vi "Main.vi"() -> ()   [LabVIEW 2014]
uses:
  <vilib>/measure/mamon.llb/Waveform Peak Detection for 1 Chan.vi
  <vilib>/measure/NI_MAPro.lvlib
panel:
  in  "Points to average":i32=50
  out "Czułość fazowa":dbl format="%#_3e"
  in  "Licz":bool
  in  "delta L [um]":dbl
  in  "L [mm]":dbl
  in  "OK Button":bool
  out "output array":dbl[](array[numeric])
  out "Locations":dbl[](array[numeric]) format="%.2p"
  in  "Reset ZOOM":bool
  out "Licznik pików":i32
  in  "stop":bool
  in  "maksimum":i32
  in  "długość przedziału":i32=100
  in  "początek przedziału":i32
  in  "próg dla maksimum":dbl format="%.2p"
  out "Waveform Graph":waveform(dbl)(graph)
  in  "file path (dialog if empty)":path
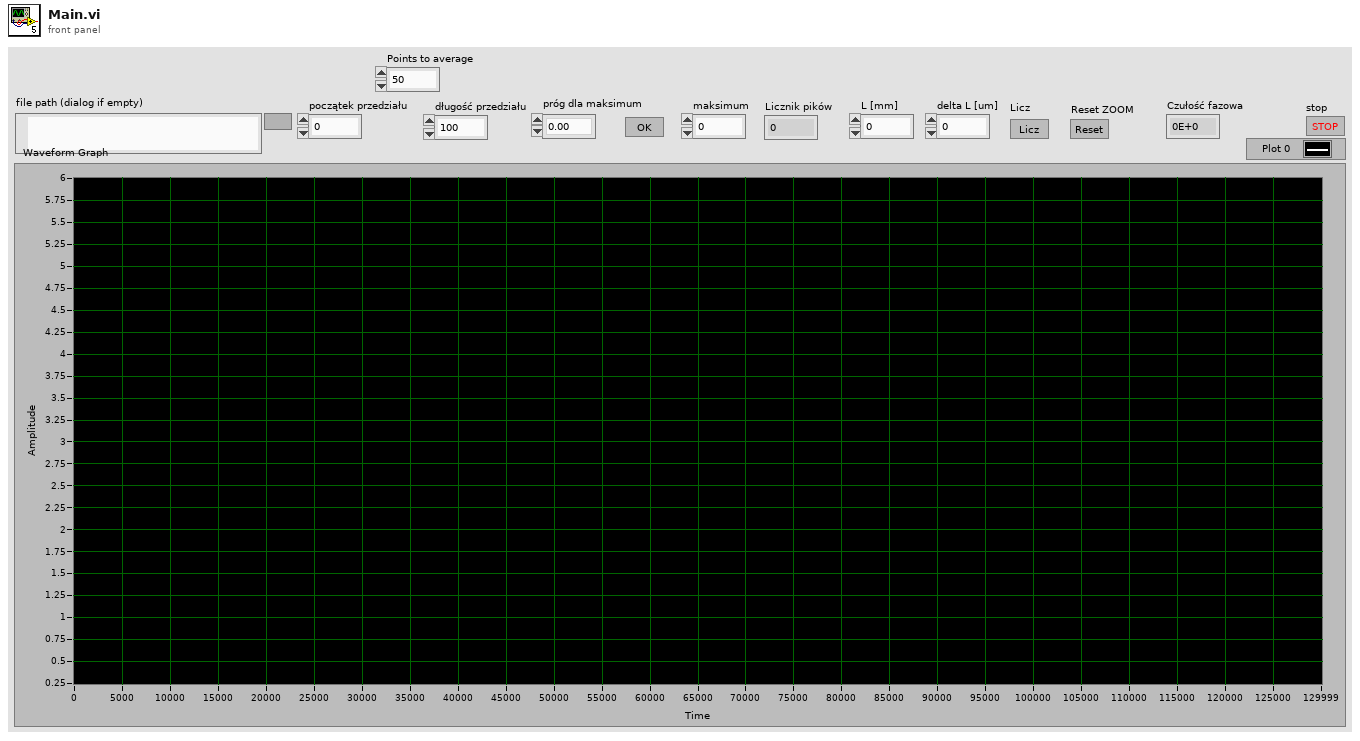
[diagram p1: front panel]
types:
  T1 = typedef "eventvkey.ctl" = enum16{"ASCII", "Enter", "Return", "Shift", "Ctrl", "Alt", "Cmd", "Opt", "Caps", "NumLock", "Clear", "Break", "Up", "Down", "Left", "Right", "Insert", "Delete", "Home", "End", "PageUp", "PageDown", "Escape", "Help", "Pause", "ScrollLock", "F1", "F2", "F3", "F4", "F5", "F6", "F7", "F8", "F9", "F10", "F11", "F12", "F13", "F14", "F15", "F16", "F17", "F18", "F19", "F20", "F21", "F22", "F23", "F24", "Play", "VolumeUp", "VolumeDown", "Mute", "Two Byte Char"}
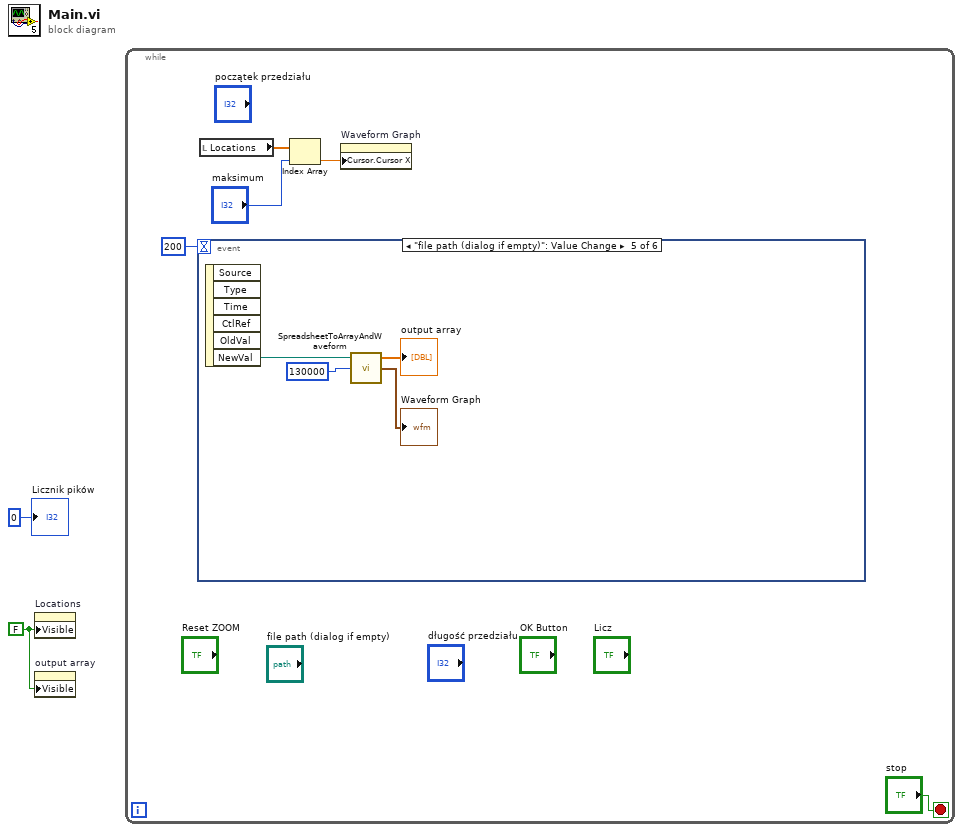
[diagram p0: block diagram]
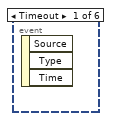
[diagram p2: hidden frame]
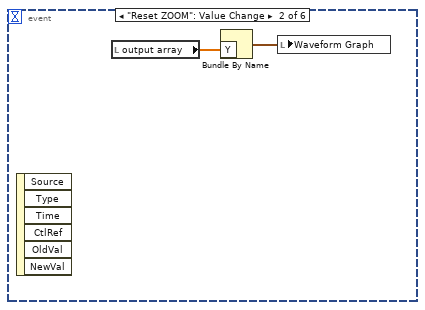
[diagram p3: hidden frame]
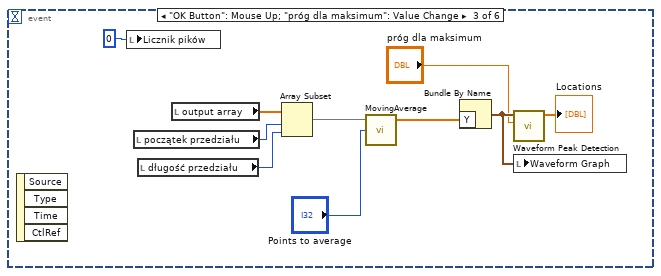
[diagram p4: hidden frame]
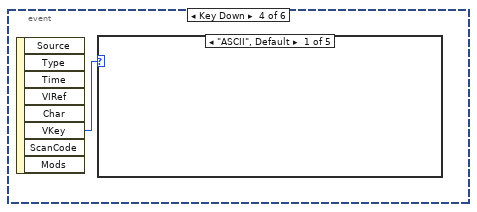
[diagram p5: hidden frame]
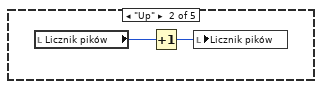
[diagram p6: hidden frame]
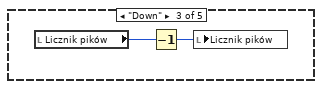
[diagram p7: hidden frame]
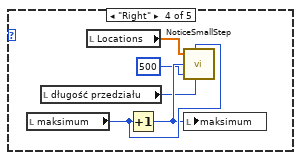
[diagram p8: hidden frame]
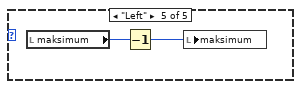
[diagram p9: hidden frame]
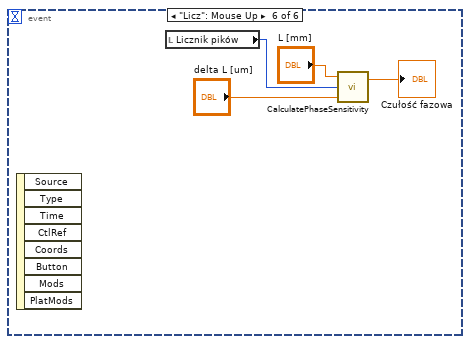
[diagram p10: hidden frame]
diagram:
  w2 = FALSE ("Visible")
  n1 = property on="Locations" class="Arr (strict)"("Visible"=w2) -> ()  [unwired: 2 in, 2 out]
  n2 = property on="output array" class="Arr (strict)"("Visible"=w2) -> ()  [unwired: 2 in, 2 out]
  n3 = while {
    stop <- "stop" stop-if-true
    n4 = event shown="[4] \"file path (dialog if empty)\": Value Change" {
      selector: _ -> [_ _ _ _ _ _]
      dyn-events: _ -> [_ _ _ _ _ _]
      timeout: 200 -> [_ _ _ _ _ _]
      event Timeout {
        n5 = event-data() -> ()  [unwired: 1 in, 3 out]
      }
      event "Reset ZOOM": Value Change {
        n6 = event-data() -> ()  [unwired: 1 in, 6 out]
        n7 = local read "output array"() -> (w9:dbl[])
        n8 = Bundle By Name("Y"=w9) -> (w8:waveform(dbl))  [unwired: 1 in]
        n9 = local write "Waveform Graph"(w8) -> ()
      }
      event "OK Button": Mouse Up; "próg dla maksimum": Value Change {
        n10 = event-data() -> ()  [unwired: 1 in, 4 out]
        n11 = local write "Licznik pików"(0 ("Licznik pików")) -> ()
        n12 = local read "początek przedziału"() -> (w16:i32)
        n13 = local read "długość przedziału"() -> (w15:i32)
        n14 = local read "output array"() -> (w14:dbl[])
        n15 = Array Subset(array=w14, index=w16, length=w15) -> (w13:dbl[])
        n16 = call "MovingAverage.vi"("Points to average"="Points to average", "Input array"=w13) -> ("Output array"=w12:dbl[])  [unwired: 2 in, 1 out]
        n17 = Bundle By Name("Y"=w12) -> (w19:waveform(dbl))  [unwired: 1 in]
        n18 = call-poly <vilib>:"Waveform Peak Detection.vi"("threshold"="próg dla maksimum", "Signal In"=w19) -> ("Locations"=→"Locations":dbl[])  [unwired: 5 in, 4 out]
        n19 = local write "Waveform Graph"(w19) -> ()
      }
      event Key Down {
        n20 = event-data() -> ("VKey"=w20:T1)  [unwired: 1 in, 7 out]
        n21 = case shown="\"ASCII\", Default" w20 {
          frame "ASCII", Default {
          }
          frame "Up" {
            n22 = local read "Licznik pików"() -> (w22:i32)
            n23 = Increment(x=w22) -> (x+1=w21:i32)
            n24 = local write "Licznik pików"(w21) -> ()
          }
          frame "Down" {
            n25 = local read "Licznik pików"() -> (w24:i32)
            n26 = Decrement(x=w24) -> (x-1=w23:i32)
            n27 = local write "Licznik pików"(w23) -> ()
          }
          frame "Right" {
            n28 = local read "maksimum"() -> (w29:i32)
            n29 = local read "długość przedziału"() -> (w25:i32)
            n30 = local read "Locations"() -> (w26:dbl[])
            n31 = Increment(x=w29) -> (x+1=w28:i32)
            n32 = call "NoticeSmallStep.vi"("array"=w26, "previous index"=w29, "next index"=w28, "step size"=500, "range size"=w25) -> ()  [unwired: 1 in]
            n33 = local write "maksimum"(w28) -> ()
          }
          frame "Left" {
            n34 = local read "maksimum"() -> (w31:i32)
            n35 = Decrement(x=w31) -> (x-1=w30:i32)
            n36 = local write "maksimum"(w30) -> ()
          }
        }
      }
      event "file path (dialog if empty)": Value Change {
        n37 = event-data() -> ("NewVal"=w32:path)  [unwired: 1 in, 5 out]
        n38 = call "SpreadsheetToArrayAndWaveform.vi"("dimension size"=130000, "file path (dialog if empty)"=w32) -> ("Waveform Graph"=→"Waveform Graph":waveform(dbl), "output array"=→"output array":dbl[])  [unwired: 2 in]
      }
      event "Licz": Mouse Up {
        n39 = event-data() -> ()  [unwired: 1 in, 8 out]
        n40 = local read "Licznik pików"() -> (w37:i32)
        n41 = call "CalculatePhaseSensitivity.vi"("delta L"="delta L [um]", "n"=w37, "L"="L [mm]") -> ("Czułość fazowa"=→"Czułość fazowa":dbl)  [unwired: 1 in]
      }
    }
    n42 = local read "Locations"() -> (w3:dbl[])
    n43 = Index Array(array=w3, index="maksimum") -> (element=w6:dbl)
    n44 = property on="Waveform Graph" class="WFGraph (strict)"("Cursor.Cursor X"=w6) -> ()  [unwired: 2 in, 2 out]
  }
  "Licznik pików" <- 0 ("Licznik pików")
